vi "Send_Command_Ref.vi"(8 "error in":errorcluster, 10 "command":string="PING", 11 "TCP session in":refnum<k5>) -> (0 "error out":errorcluster, 2 "Data":T1, 3 "TCP session out":refnum<k5>)   [LabVIEW 2023]
uses:
  SubVIs/Controls/redis-data.ctl
  SubVIs/Controls/redis-type.ctl
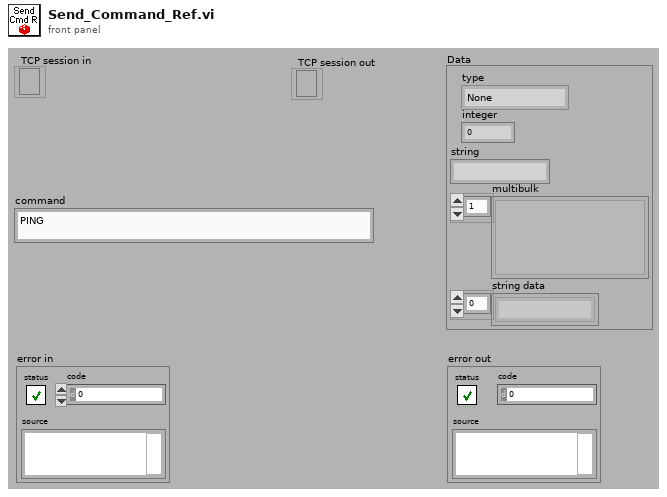
[diagram p1: front panel]
types:
  T1 = typedef "redis-data.ctl" = cluster{"type":enum16{"None", "Error", "Status", "Nil", "Integer", "String", "Multibulk"}, "integer":i64, "string":string, "multibulk":variant[], "string data":string[]}
  T2 = typedef "redis-type.ctl" = enum16{"None", "Error", "Status", "Nil", "Integer", "String", "Multibulk"}
  T3 = cluster{"integer":i64, "string":string, "multibulk":variant[]}
  T4 = typedef "redis-reply.ctl" = cluster{"integer":i64, "string":string, "multibulk":variant[]}
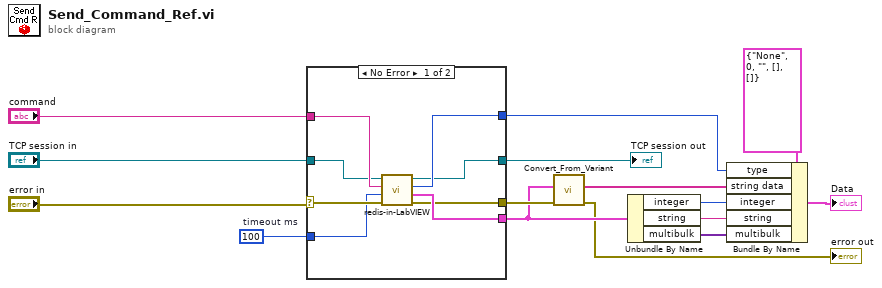
[diagram p0: block diagram]
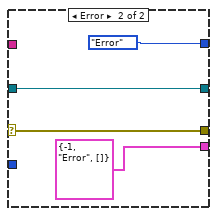
[diagram p2: hidden frame]
diagram:
  w15 = 100  # timeout ms
  n1 = case shown="No Error" "error in" {
    selector: "error in" -> [w22 w27]
    tunnel: [w23 redis-type."Error" ("reply type")] -> w12
    tunnel: [w19 T3 {"integer"=-1, "string"="Error", "multibulk"=[]} ("reply")] -> w5
    tunnel: [w18 w27] -> w6
    tunnel: w15 -> [w21 _]
    tunnel: "command" -> [w20 _]
    tunnel: "TCP session in" -> [w17 w24]
    tunnel: [w16 w24] -> w1
    frame No Error {
      n2 = call "redis-in-LabVIEW.vi"("Error in"=w22, "Timeout ms"=w21, "Command"=w20, "TCP in"=w17) -> ("Error out"=w18:errorcluster, "redis reply"=w19:T4, "reply type"=w23:T2, "TCP out"=w16:refnum<k5>)
    }
    frame Error {
    }
  }
  "TCP session out" <- w1
  n3 = call "Convert_From_Variant.vi"("error in"=w6, "Data in"=w5) -> ("error out"=→"error out":errorcluster, "String data out"=w3:string[])  [unwired: 8 in]
  n4 = Unbundle By Name(w5) -> ("integer"=w11:i64, "string"=w10:string, "multibulk"=w9:variant[])
  n5 = Bundle By Name(cluster=T1 {"type"=enum."None", "integer"=0, "string"="", "multibulk"=[], "string data"=[]} ("Data"), "type"=w12, "string data"=w3, "integer"=w11, "string"=w10, "multibulk"=w9) -> (→"Data":T1)
